vi "BackMapGlobalV2.2.vi"() -> ()   [LabVIEW 2014]
panel:
  in  "BackMap":i32[][](array[numeric])
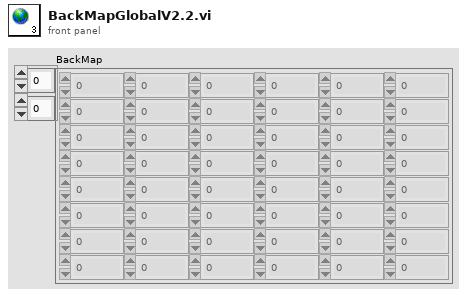
[diagram p1: front panel]
diagram:
